vi "Modified Read From SGL File.vi"(8 "error in (no error)":errorcluster, 9 "start of read offset (bytes:0)":i32, 11 "file path (dialog if empty)":path) -> (0 "error out":errorcluster, 1 "1D array":sgl[](array[numeric]) format="%.3f", 2 "2D array":sgl[][](array[numeric]) format="%.3f", 3 "new file path (Not A Path if cancelled)":path, 4 "EOF?":bool, 5 "mark after read (bytes)":i32)   [LabVIEW 2015]
doc: "Reads a 2D or 1D array of data from a byte stream file of single-precision numbers (SGL). The VI opens the file beforehand and closes it afterwards. You can use this VI to read scaled data acquired from data acquisition VIs and written to a file with Write To SGL File.\n\nfile path is the path name of the file. If file path is empty (default value) or is Not A Path, the VI displays a File dialog box from which you can select a file. Error 43 occurs if the user cancels the dialog. \n\n¥ To read the entire file into 1D array, set 1D count <0 (default); you can leave 2D number of rows unwired.\n¥ To read N elements into 1D array, set 1D count =N and leave 2D number of rows wired or set to 0.\n¥ To read the entire file into 2D array, set 2D number of rows <0 and 2D number of columns =N >0. The VI calculates the number of rows as the integer part of file size/N.\n¥ To read M rows and N columns into 2D array, set 2D number of rows =M and 2D number of columns =N.\n\nstart of read offset is the position in the file, measured in bytes, at which the VI begins reading.\n\nnew file path is the path of the file from which the VI read data. You can use this output to determine the path of a file that you open using dialog. new file path returns Not A Path if the user selects Cancel from the dialog box.\n\n2D array contains the single precision numbers read from the file if 2D number of columns is >0 and 2D number of rows is <0 (meaning read the entire file) or >0 (read the the specified number of rows) ; otherwise, this output is empty.\n\n1D array contains the single precision numbers read from the file if 1D count is <0 (meaning read the entire file) or 2D number of rows =0 and 1D count is >0 (meaning read the specified number of samples); otherwise, this output is empty.\n\nmark after read is the location of the file mark after the read; it points to the byte in the file following the last byte read.\n\nEOF? is TRUE if you attempt to read past the end of file.\n\nRevisions:\n21 Oct 93: changes incorporated to read entire file (default to read entire file as 1D array); cosmetic changes.\n12 May 94: documentation changes."
panel:
  in  "prompt":string="Choose file to read."
  in  "instructions":string="* To read the entire file into 1D array, set 1D count <0 (default); you can leave 2D number of rows unwired.\n* To read N elements into 1D array, set 1D count =N and leave 2D number of rows wired or set to 0.\n* To read the entire file into 2D array, set 2D number of rows <0 and 2D number of columns =N >0.  The VI calculates the number of rows as the integer part of file size/N.\n* To read M rows and N columns into 2D array, set 2D number of rows =M and 2D number of columns =N."
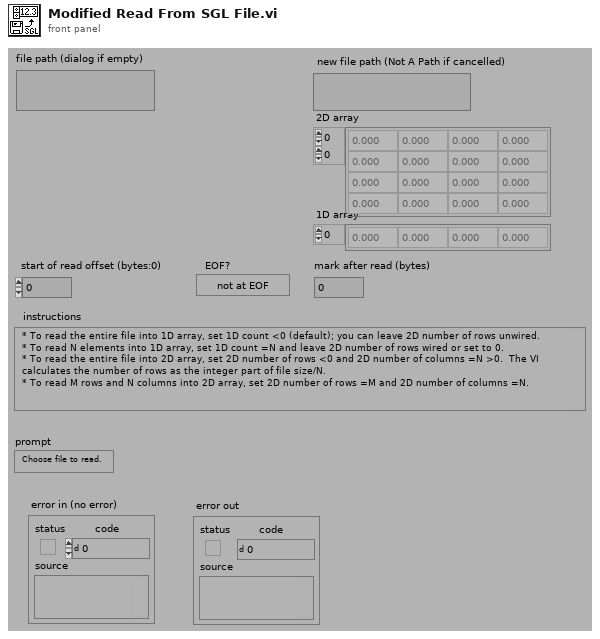
[diagram p1: front panel]
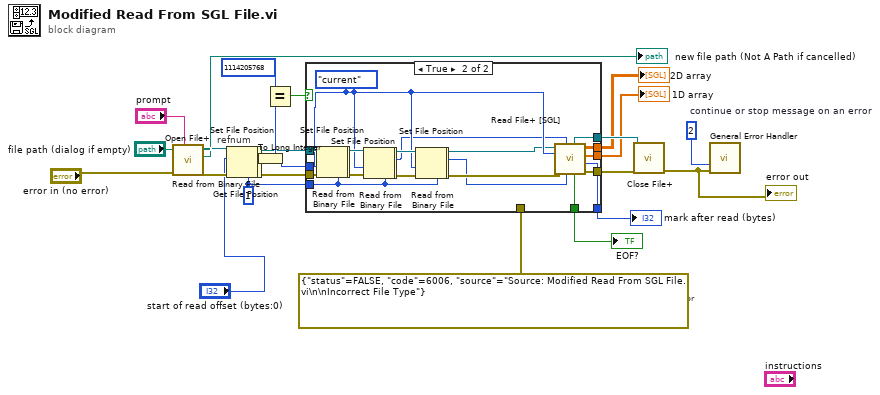
[diagram p0: block diagram]
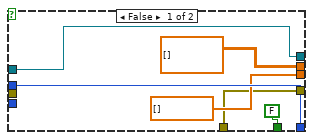
[diagram p2: hidden frame]
diagram:
  w11 = 1 ("count")
  w27 = u16 2  # continue or stop message on an error
  # "error"
  # "refnum"
  n1 = call <vilib>:"Open File+.vi"("prompt"="prompt", "error in (not an error)"="error in (no error)", "file path (\" \")"="file path (dialog if empty)") -> ("error out"=w17:errorcluster, "file path"=→"new file path (Not A Path if cancelled)":path, "refnum"=w18:refnum<file>)  [unwired: 3 in, 3 out]
  n2 = Set File Position(offset (in bytes) (0)="start of read offset (bytes:0)", refnum=w18, error in=w17) -> (refnum out=w5:refnum<file>, error out=w4:errorcluster)  [unwired: 1 out]
  n3 = Read from Binary File(5:w11, 8:w4, 11:w5) -> (0:w2:errorcluster, 2:w16:i32, 3:w3:refnum<file>)  [unwired: 4 out]
  n4 = Get File Position(4:w2, 7:w3) -> (0:w12:errorcluster, 2:w1:i64, 3:w13:refnum<file>)
  n5 = To Long Integer(number=w1) -> (32bit integer=w9:i32)
  n6 = Equal?(x=1114205768, y=w16) -> (x = y?=w15:bool)
  n7 = case shown="True" w15 {
    tunnel: [w29 w58] -> w26
    tunnel: [w34 w57] -> w25
    tunnel: [FALSE ("EOF?") w56] -> w24
    tunnel: [w30 w55] -> w23
    tunnel: [sgl[] [] ("1D data") w54] -> w22
    tunnel: [sgl[][] [] ("2D data") w53] -> w21
    tunnel: w13 -> [w30 w52]
    tunnel: w12 -> [_ w51]
    tunnel: w11 -> [_ w46]
    tunnel: w9 -> [w34 _]
    tunnel: errorcluster {"status"=FALSE, "code"=6006, "source"="Source: Modified Read From SGL File.vi\n\nIncorrect File Type"} ("error out") -> [w29 _]
    frame False {
    }
    frame True {
      w45 = enum16{"start", "end", "current"}."current" ("pos mode (0:2)")
      n8 = Set File Position(refnum=w52, from (0:start)=w45, error in=w51) -> (refnum out=w36:refnum<file>, error out=w35:errorcluster)  [unwired: 1 out]
      n9 = Read from Binary File(5:w46, 8:w35, 11:w36) -> (0:w50:errorcluster, 3:w48:refnum<file>)  [unwired: 5 out]
      n10 = Set File Position(refnum=w48, from (0:start)=w45, error in=w50) -> (refnum out=w38:refnum<file>, error out=w37:errorcluster)  [unwired: 1 out]
      n11 = Read from Binary File(5:w46, 8:w37, 11:w38) -> (0:w49:errorcluster, 2:w41:i32, 3:w47:refnum<file>)  [unwired: 4 out]
      n12 = Set File Position(refnum=w47, from (0:start)=w45, error in=w49) -> (refnum out=w40:refnum<file>, error out=w39:errorcluster)  [unwired: 1 out]
      n13 = Read from Binary File(5:w46, 8:w39, 11:w40) -> (0:w43:errorcluster, 2:w42:i32, 3:w44:refnum<file>)  [unwired: 4 out]
      n14 = call <vilib>:"Read File+ [SGL].vi"("2D number of columns/1D count"=w42, "2D number of rows"=w41, "error in (no error)"=w43, "pos mode (rel. to current:2)"=w45, "refnum"=w44) -> ("error out"=w58:errorcluster, "mark after read (bytes)"=w57:i32, "1D data"=w54:sgl[], "2D data"=w53:sgl[][], "EOF?"=w56:bool, "dup refnum"=w55:refnum<file>)  [unwired: 1 in]
    }
  }
  "1D array" <- w22
  "mark after read (bytes)" <- w25
  "EOF?" <- w24
  "2D array" <- w21
  n15 = call <vilib>:"Close File+.vi"("error in (no error)"=w26, "refnum"=w23) -> ("error out"=w6:errorcluster)  [unwired: 5 out]
  "error out" <- w6
  n16 = call <vilib>:"General Error Handler.vi"("type of dialog (OK msg:1)"=w27, "error in (no error)"=w6) -> ()  [unwired: 1 in, 13 out]
